vi "TxBfrPkt - Init Packet Page.vi"(6 "Tx Buffered Data Packet Refs":T1, 8 "error in (no error)":errorcluster, 11 "Node Ptr In":T2 format="%.0x") -> (0 "error out":errorcluster, 3 "Node Ptr Out":T2 format="%.0x")   [LabVIEW 2019, in "UDP-Custom-Device System Explorer.lvlib"]
uses:
  UDP-Custom-Device System Explorer.lvlib
  <vilib>/NI VeriStand/Custom Device API/Custom Device Item Ref.ctl
  Types/Page References/Refs - Tx Buffered Data Packet Page.ctl
  Shared/Types/Shared - Transmit Buffer Options.ctl
  Shared/Types/Shared - Transmit Sim Options.ctl
  <vilib>/NI VeriStand/Custom Device API/Custom Device API.lvlib
  Property Accessors/Shared Packet Accessors.lvlib
  Property Accessors/Buffered Data Packet.lvlib
  Property Accessors/Tx Packet Accessors.lvlib
  Shared/UDP-Custom-Device Shared.lvlib
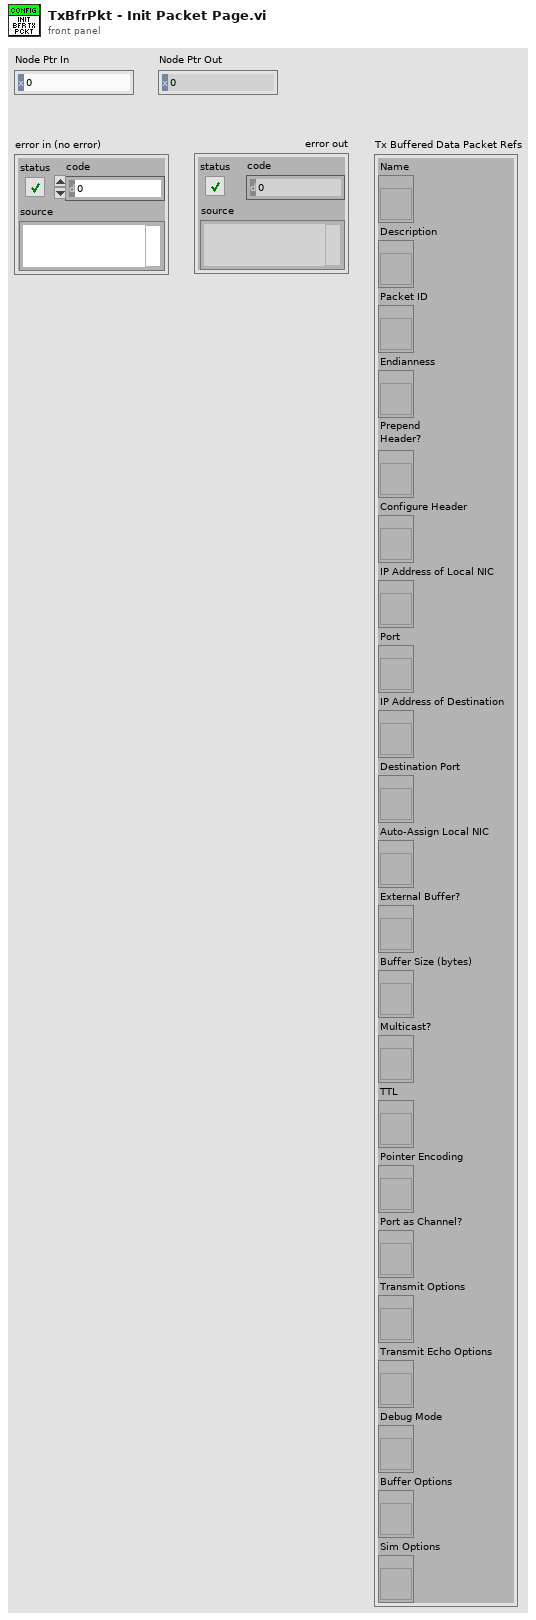
[diagram p1: front panel]
types:
  T1 = typedef "UDP-Custom-Device System Explorer.lvlib/Refs - Tx Buffered Data Packet Page.ctl" = cluster{"Name":refnum<vi>, "Description":refnum<vi>, "Packet ID":refnum<vi>, "Endianness":refnum<vi>, "Prepend\nHeader?":refnum<vi>, "Configure Header":refnum<vi>, "IP Address of Local NIC":refnum<vi>, "Port":refnum<vi>, "IP Address of Destination":refnum<vi>, "Destination Port":refnum<vi>, "Auto-Assign Local NIC":refnum<vi>, "External Buffer?":refnum<vi>, "Buffer Size (bytes)":refnum<vi>, "Multicast?":refnum<vi>, "TTL":refnum<vi>, "Pointer Encoding":refnum<vi>, "Port as Channel?":refnum<vi>, "Transmit Options":refnum<vi>, "Transmit Echo Options":refnum<vi>, "Debug Mode":refnum<vi>, "Buffer Options":refnum<vi>, "Sim Options":refnum<vi>}
  T2 = typedef "Custom Device API.lvlib/Custom Device Item Ref.ctl" = u64
  T3 = typedef "UDP-Custom-Device Shared.lvlib/Shared - Transmit Sim Options.ctl" = enum16{"No Simulation", "Counter", "Full Buffer", "FIFO Test", "FIFO + Port Test"}
  T4 = typedef "UDP-Custom-Device Shared.lvlib/Shared - Transmit Buffer Options.ctl" = enum16{"Static Buffer", "FIFO Buffer", "FIFO Buffer + Port"}
  T5 = enum8{"Enabled", "Disabled", "Disabled and Grayed Out"}
  T6 = typedef "UDP-Custom-Device Shared.lvlib/Shared - Transmit Echo Options.ctl" = enum16{"PCL Reset", "Counter", "Mirror"}
  T7 = typedef "UDP-Custom-Device Shared.lvlib/Shared - Pointer Encoding.ctl" = enum16{"Direct Encoding", "Conversion Encoding"}
  T8 = typedef "UDP-Custom-Device Shared.lvlib/Shared - Transmit Flag Options.ctl" = enum16{"Always", "One-Shot", "Toggle"}
  T9 = typedef "Custom Device API.lvlib/Custom Device Item Info.ctl" = cluster{"Name":string, "Is Channel":bool, "GUID":string, "Is Waveform":bool}
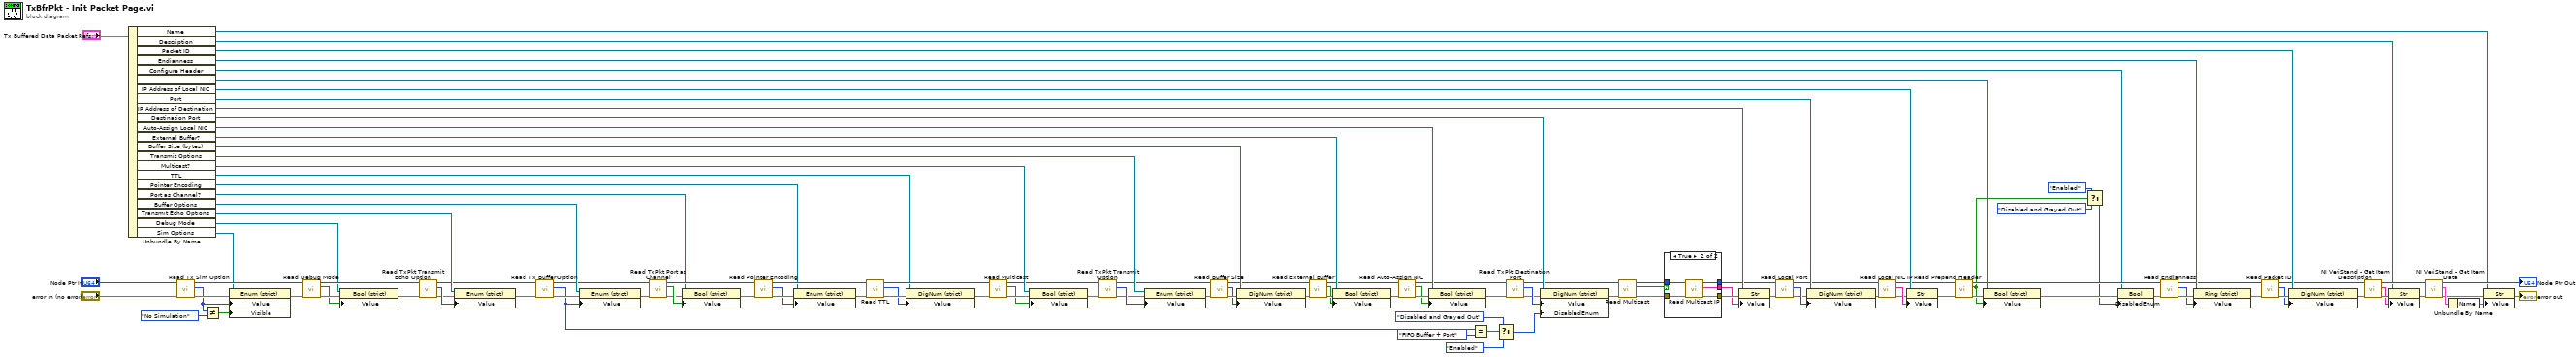
[diagram p0: block diagram]
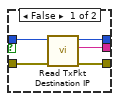
[diagram p2: hidden frame]
diagram:
  n1 = Unbundle By Name("Tx Buffered Data Packet Refs") -> ("Name"=w114:refnum<vi>, "Description"=w113:refnum<vi>, "Packet ID"=w112:refnum<vi>, "Endianness"=w105:refnum<vi>, "Configure Header"=w94:refnum<vi>, "Prepend\nHeader?"=w102:refnum<vi>, "IP Address of Local NIC"=w92:refnum<vi>, "Port"=w88:refnum<vi>, "IP Address of Destination"=w82:refnum<vi>, "Destination Port"=w79:refnum<vi>, "Auto-Assign Local NIC"=w75:refnum<vi>, "External Buffer?"=w71:refnum<vi>, "Buffer Size (bytes)"=w69:refnum<vi>, "Transmit Options"=w61:refnum<vi>, "Multicast?"=w55:refnum<vi>, "TTL"=w53:refnum<vi>, "Pointer Encoding"=w45:refnum<vi>, "Port as Channel?"=w40:refnum<vi>, "Buffer Options"=w31:refnum<vi>, "Transmit Echo Options"=w29:refnum<vi>, "Debug Mode"=w25:refnum<vi>, "Sim Options"=w8:refnum<vi>)
  n2 = call "Read Tx Sim Option.vi"("error in (no error)"="error in (no error)", "Node Ptr"="Node Ptr In") -> ("error out"=w7:errorcluster, "Sim Option"=w5:T3, "Node Ptr out"=w10:T2)  [unwired: 7 in]
  n3 = Not Equal?(x=w5, y=Shared_-_Transmit_Sim_Options."No Simulation") -> (x != y?=w3:bool)
  n4 = property class="Enum (strict)"(reference=w8, error in=w7, "Value"=w5, "Visible"=w3) -> (error out=w6:errorcluster)  [unwired: 1 out]
  n5 = call "Read Debug Mode.vi"("error in (no error)"=w6, "Node Ptr"=w10) -> ("error out"=w24:errorcluster, "Debug Mode"=w22:bool, "Node Ptr out"=w27:T2)  [unwired: 7 in]
  n6 = property class="Bool (strict)"(reference=w25, error in=w24, "Value"=w22) -> (error out=w23:errorcluster)  [unwired: 1 out]
  n7 = call "Read TxPkt Transmit Echo Option.vi"("error in (no error)"=w23, "Node Ptr"=w27) -> ("error out"=w26:errorcluster, "Transmit Echo Options"=w28:T6, "Node Ptr out"=w21:T2)  [unwired: 7 in]
  n8 = property class="Enum (strict)"(reference=w29, error in=w26, "Value"=w28) -> (error out=w20:errorcluster)  [unwired: 1 out]
  n9 = call "Read Tx Buffer Option.vi"("error in (no error)"=w20, "Node Ptr"=w21) -> ("error out"=w19:errorcluster, "Buffer Option"=w14:T4, "Node Ptr out"=w18:T2)  [unwired: 7 in]
  n10 = property class="Enum (strict)"(reference=w31, error in=w19, "Value"=w14) -> (error out=w30:errorcluster)  [unwired: 1 out]
  n11 = call "Read TxPkt Port as Channel.vi"("error in (no error)"=w30, "Node Ptr"=w18) -> ("error out"=w38:errorcluster, "Port as Channel"=w39:bool, "Node Ptr out"=w41:T2)  [unwired: 7 in]
  n12 = property class="Bool (strict)"(reference=w40, error in=w38, "Value"=w39) -> (error out=w37:errorcluster)  [unwired: 1 out]
  n13 = call "Read Pointer Encoding.vi"("error in (no error)"=w37, "Node Ptr"=w41) -> ("error out"=w43:errorcluster, "Pointer Encoding"=w42:T7, "Node Ptr out"=w46:T2)  [unwired: 7 in]
  n14 = property class="Enum (strict)"(reference=w45, error in=w43, "Value"=w42) -> (error out=w44:errorcluster)  [unwired: 1 out]
  n15 = call "Read TTL.vi"("error in (no error)"=w44, "Node Ptr"=w46) -> ("error out"=w57:errorcluster, "TTL"=w52:u16, "Node Ptr out"=w59:T2)  [unwired: 7 in]
  n16 = property class="DigNum (strict)"(reference=w53, error in=w57, "Value"=w52) -> (error out=w58:errorcluster)  [unwired: 1 out]
  n17 = call "Read Multicast.vi"("error in (no error)"=w58, "Node Ptr"=w59) -> ("error out"=w56:errorcluster, "Multicast"=w54:bool, "Node Ptr out"=w36:T2)  [unwired: 7 in]
  n18 = property class="Bool (strict)"(reference=w55, error in=w56, "Value"=w54) -> (error out=w35:errorcluster)  [unwired: 1 out]
  n19 = call "Read TxPkt Transmit Option.vi"("error in (no error)"=w35, "Node Ptr"=w36) -> ("error out"=w33:errorcluster, "Transmit Options"=w34:T8, "Node Ptr out"=w32:T2)  [unwired: 7 in]
  n20 = property class="Enum (strict)"(reference=w61, error in=w33, "Value"=w34) -> (error out=w60:errorcluster)  [unwired: 1 out]
  n21 = call "Read Buffer Size.vi"("error in (no error)"=w60, "Node Ptr"=w32) -> ("error out"=w63:errorcluster, "Buffer Size"=w62:u32, "Node Ptr out"=w68:T2)  [unwired: 7 in]
  n22 = property class="DigNum (strict)"(reference=w69, error in=w63, "Value"=w62) -> (error out=w66:errorcluster)  [unwired: 1 out]
  n23 = call "Read External Buffer.vi"("error in (no error)"=w66, "Node Ptr"=w68) -> ("error out"=w65:errorcluster, "External Buffer"=w64:bool, "Node Ptr out"=w67:T2)  [unwired: 7 in]
  n24 = property class="Bool (strict)"(reference=w71, error in=w65, "Value"=w64) -> (error out=w70:errorcluster)  [unwired: 1 out]
  n25 = call "Read Auto-Assign NIC.vi"("error in (no error)"=w70, "Node Ptr"=w67) -> ("error out"=w74:errorcluster, "Auto-Assign NIC"=w73:bool, "Node Ptr out"=w72:T2)  [unwired: 7 in]
  n26 = property class="Bool (strict)"(reference=w75, error in=w74, "Value"=w73) -> (error out=w76:errorcluster)  [unwired: 1 out]
  n27 = Equal?(x=w14, y=Shared_-_Transmit_Buffer_Options."FIFO Buffer + Port") -> (x = y?=w12:bool)
  n28 = Select(t=T5."Disabled and Grayed Out" ("Disabled"), s=w12, f=T5."Enabled" ("Disabled")) -> (s? t:f=w15:T5)
  n29 = call "Read TxPkt Destination Port.vi"("error in (no error)"=w76, "Node Ptr"=w72) -> ("error out"=w77:errorcluster, "Destination Port"=w78:u16, "Node Ptr out"=w51:T2)  [unwired: 7 in]
  n30 = property class="DigNum (strict)"(reference=w79, error in=w77, "Value"=w78, "DisabledEnum"=w15) -> (error out=w49:errorcluster)  [unwired: 1 out]
  n31 = call "Read Multicast.vi"("error in (no error)"=w49, "Node Ptr"=w51) -> ("error out"=w48:errorcluster, "Multicast"=w47:bool, "Node Ptr out"=w50:T2)  [unwired: 7 in]
  n32 = case shown="True" w47 {
    tunnel: [w129 w130] -> w83
    tunnel: [w128 w131] -> w81
    tunnel: [w127 w132] -> w80
    tunnel: w50 -> [w126 w134]
    tunnel: w48 -> [w125 w133]
    frame False {
      n33 = call "Read TxPkt Destination IP.vi"("error in (no error)"=w125, "Node Ptr"=w126) -> ("error out"=w129:errorcluster, "Destination IP"=w128:string, "Node Ptr out"=w127:T2)  [unwired: 7 in]
    }
    frame True {
      n34 = call "Read Multicast IP.vi"("error in (no error)"=w133, "Node Ptr"=w134) -> ("error out"=w130:errorcluster, "Multicast IP Address"=w131:string, "Node Ptr out"=w132:T2)  [unwired: 7 in]
    }
  }
  n35 = property class="Str"(reference=w82, error in=w83, "Value"=w81) -> (error out=w84:errorcluster)  [unwired: 1 out]
  n36 = call "Read Local Port.vi"("error in (no error)"=w84, "Node Ptr"=w80) -> ("error out"=w86:errorcluster, "Port"=w87:u16, "Node Ptr out"=w85:T2)  [unwired: 7 in]
  n37 = property class="DigNum (strict)"(reference=w88, error in=w86, "Value"=w87) -> (error out=w89:errorcluster)  [unwired: 1 out]
  n38 = call "Read Local NIC IP.vi"("error in (no error)"=w89, "Node Ptr"=w85) -> ("error out"=w90:errorcluster, "IP Address of Local NIC"=w91:string, "Node Ptr out"=w2:T2)  [unwired: 7 in]
  n39 = property class="Str"(reference=w92, error in=w90, "Value"=w91) -> (error out=w1:errorcluster)  [unwired: 1 out]
  n40 = call "Read Prepend Header.vi"("error in (no error)"=w1, "Node Ptr"=w2) -> ("error out"=w101:errorcluster, "Prepend Header"=w97:bool, "Node Ptr out"=w100:T2)  [unwired: 7 in]
  n41 = property class="Bool (strict)"(reference=w102, error in=w101, "Value"=w97) -> (error out=w96:errorcluster)  [unwired: 1 out]
  n42 = Select(t=T5."Enabled" ("Disabled"), s=w97, f=T5."Disabled and Grayed Out" ("Disabled")) -> (s? t:f=w93:T5)
  n43 = property class="Bool"(reference=w94, error in=w96, "DisabledEnum"=w93) -> (error out=w95:errorcluster)  [unwired: 1 out]
  n44 = call "Read Endianness.vi"("error in (no error)"=w95, "Node Ptr"=w100) -> ("error out"=w106:errorcluster, "Endianness"=w104:u16, "Node Ptr out"=w103:T2)  [unwired: 7 in]
  n45 = property class="Ring (strict)"(reference=w105, error in=w106, "Value"=w104) -> (error out=w107:errorcluster)  [unwired: 1 out]
  n46 = call "Read Packet ID.vi"("error in (no error)"=w107, "Node Ptr"=w103) -> ("error out"=w109:errorcluster, "Packet ID"=w108:i32, "Node Ptr out"=w110:T2)  [unwired: 7 in]
  n47 = property class="DigNum (strict)"(reference=w112, error in=w109, "Value"=w108) -> (error out=w111:errorcluster)  [unwired: 1 out]
  n48 = call <vilib>:"NI VeriStand - Get Item Description.vi"("error in (no error)"=w111, "Item Ref in"=w110) -> ("error out"=w121:errorcluster, "Description"=w120:string, "Item Ref out"=w118:T2)  [unwired: 7 out]
  n49 = property class="Str"(reference=w113, error in=w121, "Value"=w120) -> (error out=w119:errorcluster)  [unwired: 1 out]
  n50 = call <vilib>:"NI VeriStand - Get Item Data.vi"("error in (no error)"=w119, "Item Ref in"=w118) -> ("error out"=w122:errorcluster, "Item Info"=w123:T9, "Item Ref out"=→"Node Ptr Out":T2)  [unwired: 6 in, 1 out]
  n51 = Unbundle By Name(w123) -> ("Name"=w117:string)
  n52 = property class="Str"(reference=w114, error in=w122, "Value"=w117) -> (error out=→"error out":errorcluster)  [unwired: 1 out]
